vi "Post Sub Step WaitMoniter.vi"(10 "WaitMoniter Input":T1={"Wait Time(S)"=10.0, "Chamber Temp(Deg C)"=10.0, "Chamber Temp Tolerance(%)"=10.0, "RMS Current(A)"=10.0, "RMS Current Tolerance(%)"=10.0, "Temperature Control"=FALSE, "RMS Control"=FALSE, "RMS Current Min(A)"=48.0, "RMS Current Max(A)"=150.0, "Chamber Temp Min(Deg C)"=55.0, "Chamber Temp Max(Deg C)"=160.0, "HVPPS Current Max(A)"=-0.11, "HVPPS Control"=FALSE, "HVPPS Current(A)"=0.0} {"HVPPS Current(A)" format="%#_13g"; "HVPPS Current Max(A)" format="%#_13g"; "Chamber Temp Max(Deg C)" format="%#_13g"; "Chamber Temp Min(Deg C)" format="%#_13g"; "RMS Current Max(A)" format="%#_13g"; "RMS Current Min(A)" format="%#_13g"; "RMS Current Tolerance(%)" format="%#_13g"; "RMS Current(A)" format="%#_13g"; "Chamber Temp Tolerance(%)" format="%#_13g"; "Chamber Temp(Deg C)" format="%#_13g"; "Wait Time(S)" format="%#_13g"}, 11 "Sequence Context In":refnum<k7>) -> (0 "error out":errorcluster, 3 "Report Text":string)   [LabVIEW 2023, in "LTT_TeststandSteptypes.lvlib"]
uses:
  LTT_TeststandSteptypes.lvlib
  Control/Moniter Step Control.ctl
  HardwareAbstractionLayer_LVOOP/Power Moniter/Wait Monitor_class/Wait Monitor.lvclass
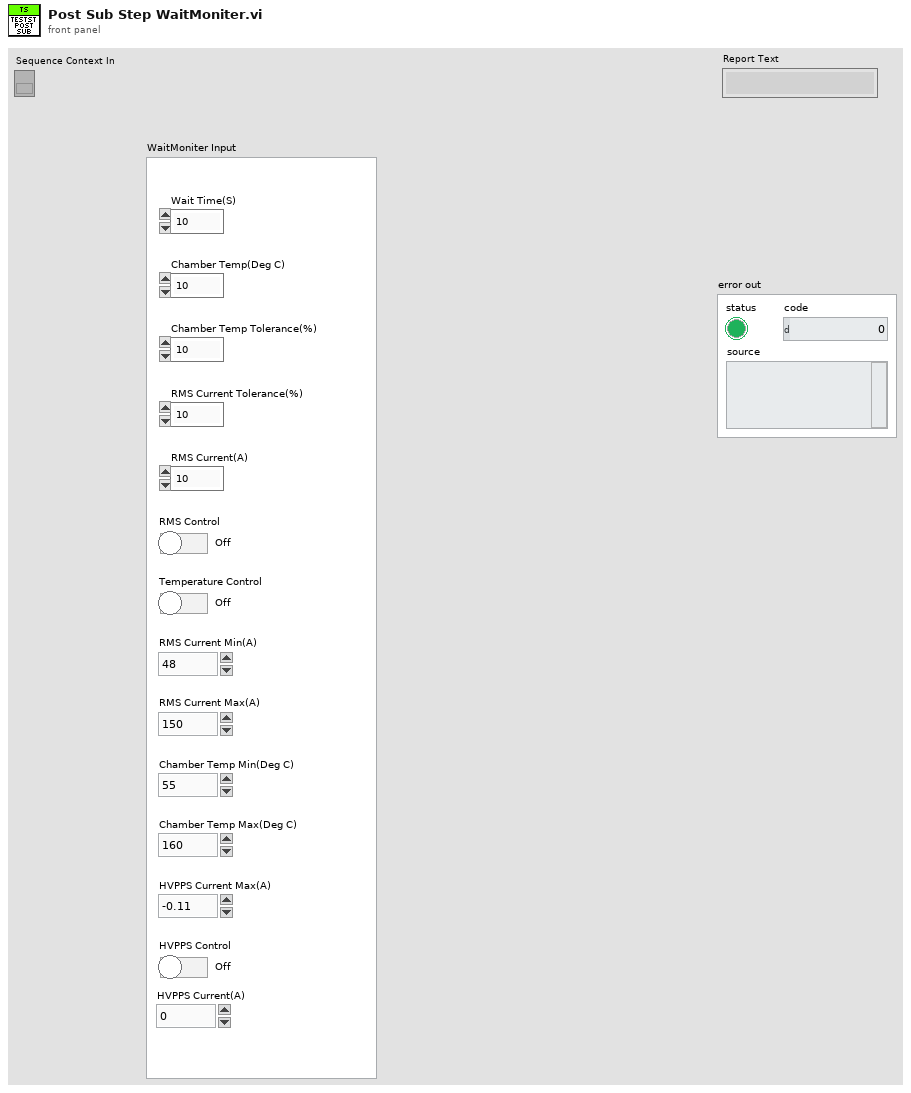
[diagram p1: front panel]
types:
  T1 = typedef "HardwareAbstractionLayer_LVOOP.lvlib/Wait Monitor.lvclass/Moniter Step Control.ctl" = cluster{"Wait Time(S)":dbl, "Chamber Temp(Deg C)":dbl, "Chamber Temp Tolerance(%)":dbl, "RMS Current(A)":dbl, "RMS Current Tolerance(%)":dbl, "Temperature Control":bool, "RMS Control":bool, "RMS Current Min(A)":dbl, "RMS Current Max(A)":dbl, "Chamber Temp Min(Deg C)":dbl, "Chamber Temp Max(Deg C)":dbl, "HVPPS Current Max(A)":dbl, "HVPPS Control":bool, "HVPPS Current(A)":dbl}
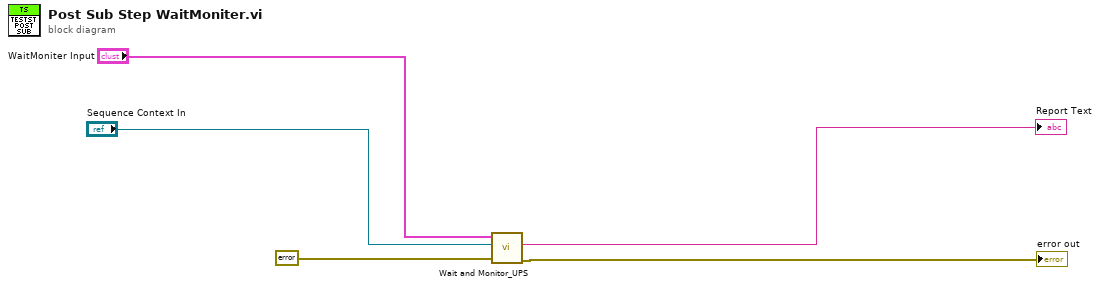
[diagram p0: block diagram]
diagram:
  n1 = call "Wait and Monitor_UPS.vi"("error in"=errorcluster {"status"=FALSE, "code"=0, "source"=""}, "Sequence Context"="Sequence Context In", "WaitMoniter Input"="WaitMoniter Input") -> ("error out"=→"error out":errorcluster, "Report Text"=→"Report Text":string)  [unwired: 6 in, 1 out]
